vi "SRC_var_globale.vi"() -> ()   [LabVIEW 2010, in "lv_04.lvlib"]
uses:
  lv_04.lvlib
panel:
  in  "Nb décimales":u16=2
  in  "Code src":string="005"
  in  "Chemin TDMS":path=path "D:/nidev/src/src.tdms"
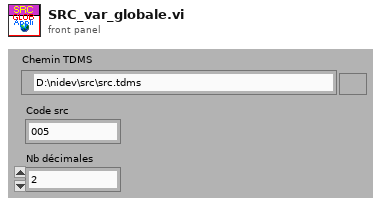
[diagram p1: front panel]
diagram:
